vi "FlatToRichcif_common_ShortVersion.vi"(5 "OutputClusterType":T1, 11 "InputCluster":T2) -> (3 "OutputCluster":T1)   [LabVIEW 2021, in "CIFCorePlugin_client.lvlib"]
uses:
  cif_common_ShortVersion_Flat.ctl
  cif_common_ShortVersion.ctl
  CIFCorePlugin_client.lvlib
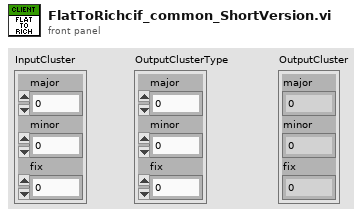
[diagram p1: front panel]
types:
  T1 = typedef "CIFCorePlugin_client.lvlib/cif_common_ShortVersion.ctl" = cluster{"major":u32, "minor":u32, "fix":u32}
  T2 = typedef "CIFCorePlugin_client.lvlib/cif_common_ShortVersion_Flat.ctl" = cluster{"major":u32, "minor":u32, "fix":u32}
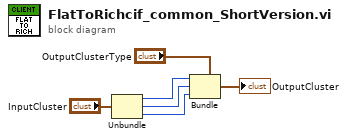
[diagram p0: block diagram]
diagram:
  n1 = Unbundle "Unbundle"("InputCluster") -> ("major"=w3:u32, "minor"=w2:u32, "fix"=w1:u32)
  n2 = Bundle "Bundle"(cluster="OutputClusterType", "major"=w3, "minor"=w2, "fix"=w1) -> (→"OutputCluster":T1)
